vi "例9.2 采集一段波形.vi"() -> ()   [LabVIEW 2012]
doc: "本VI说明了从指定设备采集有限声音采样的方式。需要使用连接至声卡的麦克风。可指定需采集的采样数、采样率、通道数和每采样比特率。"
uses:
  <vilib>/sound2/lvsound2.llb/Sound Data Format.ctl
  <vilib>/sound2/lvsound2.llb/Sampling Mode.ctl
  <vilib>/sound2/lvsound2.llb/Sound Input Read (DBL).vi
panel:
  in  "Sound Format":T1={"sample rate (S/s)"=22050.0, "number of channels"=2, "bits per sample"=16} caption="声音格式"
  in  "Device ID":u32 caption="设备ID" format="%.0x"
  out "Sound Input":waveform(dbl)[](graph) caption="采集的声音"
  in  "Number of Samples/ch":i32=10000 caption="每通道采样数"
  # "配置"
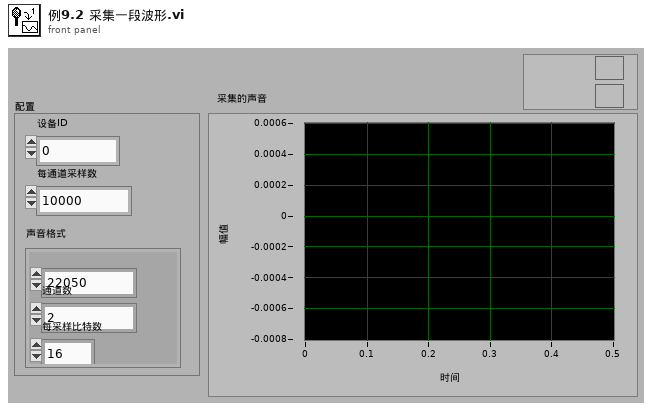
[diagram p1: front panel]
types:
  T1 = typedef "Sound Data Format.ctl" = cluster{"sample rate (S/s)":dbl, "number of channels":i32, "bits per sample":i32}
  T2 = typedef "Sampling Mode.ctl" = i32
  T3 = typedef "Sound Input Task ID.ctl" = u32
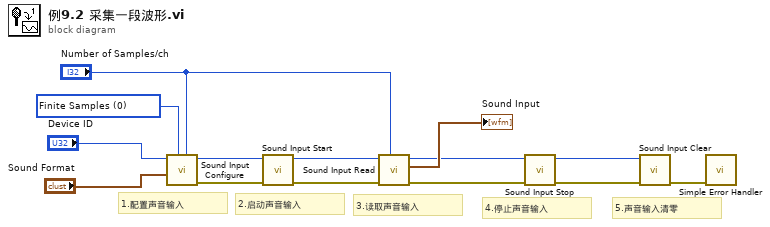
[diagram p0: block diagram]
diagram:
  w12 = T2 0 items=["Finite Samples", "Continuous Samples"] ("sample mode")
  # "5.声音输入清零"
  # "4.停止声音输入"
  # "3.读取声音输入"
  # "2.启动声音输入"
  # "1.配置声音输入"
  n1 = call <vilib>:"Sound Input Configure.vi"("number of samples/ch"="Number of Samples/ch", "sample mode"=w12, "sound format"="Sound Format", "device ID"="Device ID") -> ("error out"=w7:errorcluster, "task ID"=w8:T3)  [unwired: 6 in]
  n2 = call <vilib>:"Sound Input Start.vi"("error in (no error)"=w7, "task ID"=w8) -> ("error out"=w5:errorcluster, "task ID out"=w6:T3)  [unwired: 8 in]
  n3 = call-poly <vilib>:"Sound Input Read.vi"("number of samples/ch"="Number of Samples/ch", "error in (no error)"=w5, "task ID"=w6) -> ("error out"=w3:errorcluster, "data"=→"Sound Input":waveform(dbl)[], "task ID out"=w4:T3)  [unwired: 6 in]
  n4 = call <vilib>:"Sound Input Stop.vi"("error in (no error)"=w3, "task ID"=w4) -> ("error out"=w1:errorcluster, "task ID out"=w2:T3)  [unwired: 8 in]
  n5 = call <vilib>:"Sound Input Clear.vi"("error in (no error)"=w1, "task ID"=w2) -> ("error out"=w9:errorcluster)  [unwired: 9 in]
  n6 = call <vilib>:"Simple Error Handler.vi"("error in (no error)"=w9) -> ()  [unwired: 4 in, 5 out]
